vi "Data Storage.vi"(9 "Time Out In ms":i32=-1, 10 "Data In":u16[][](array[numeric]), 11 "Circular Buffer 2D U16 DVR Queue Circular Buffer in":refnum<class "Circular Buffer 2D U16 DVR Queue Circular Buffer.lvclass">) -> (1 "Time Out":bool, 3 "Circular Buffer 2D U16 DVR Queue Circular Buffer out":refnum<class "Circular Buffer 2D U16 DVR Queue Circular Buffer.lvclass">)   [LabVIEW 2019, in "Circular Buffer 2D U16 DVR Queue Circular Buffer.lvclass"]
uses:
  Circular Buffer 2D U16 DVR Queue Circular Buffer.lvclass
  Circular Buffer 2D U16 DVR Queue Circular Buffer.lvclass/Circular Buffer 2D U16 DVR Queue Circular Buffer.ctl
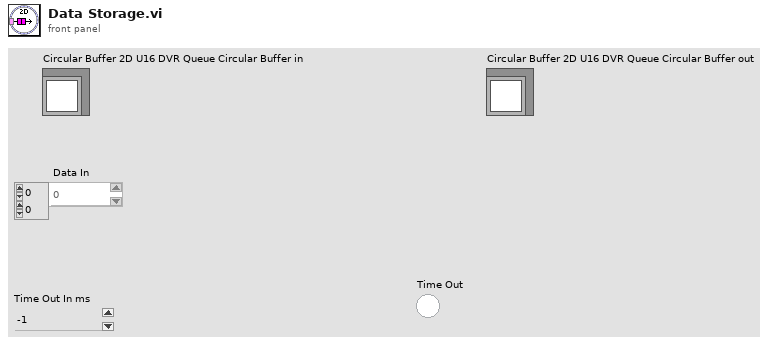
[diagram p1: front panel]
types:
  T1 = typedef "2D U16 DVR Queue.ctl" = refnum<queue>
  T2 = typedef "2D U16 DVR.ctl" = refnum<data-value>
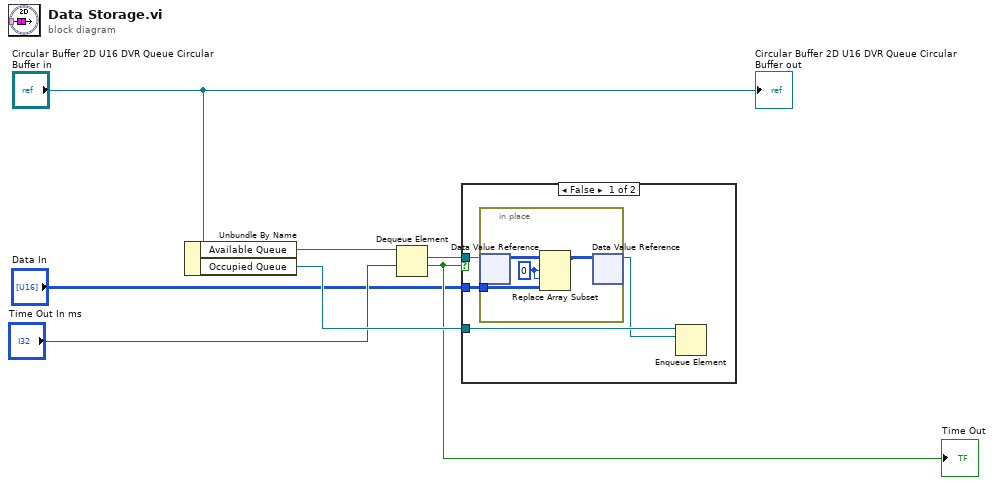
[diagram p0: block diagram]
diagram:
  n1 = Unbundle By Name("Circular Buffer 2D U16 DVR Queue Circular Buffer in") -> ("Available Queue"=w6:T1, "Occupied Queue"=w7:T1)
  n2 = Dequeue Element(queue=w6, timeout in ms (-1)="Time Out In ms") -> (element=w4:T2, timed out?=w3:bool)  [unwired: 1 in, 2 out]
  "Time Out" <- w3
  n3 = case shown="False" w3 {
    tunnel: w4 -> [w11 _]
    tunnel: w7 -> [w10 _]
    tunnel: "Data In" -> [w8 _]
    frame False {
      n4 = in-place {
        in-place-border: w8 -> [w12]
        w13 = 0 ("index (row)")
        n5 = in-place-dvr #1(w11) -> (w15:u16[][])  [unwired: 1 out]
        n6 = Replace Array Subset(array=w15, new element=w12, index (row)=w13, index (col)=w13) -> (w14:u16[][])
        n7 = in-place-dvr #1(w14) -> (w9:T2)  [unwired: 1 out]
      }
      n8 = Enqueue Element(queue=w10, element=w9) -> ()  [unwired: 2 in, 3 out]
    }
    frame True {
    }
  }
  "Circular Buffer 2D U16 DVR Queue Circular Buffer out" <- "Circular Buffer 2D U16 DVR Queue Circular Buffer in"
